vi "Convert Array from IH.vi"(1 "IH":T1) -> (0 "Array":u8[](array[numeric]))   [LabVIEW 2013, in "VRI.lvlib"]
uses:
  VRI.lvlib
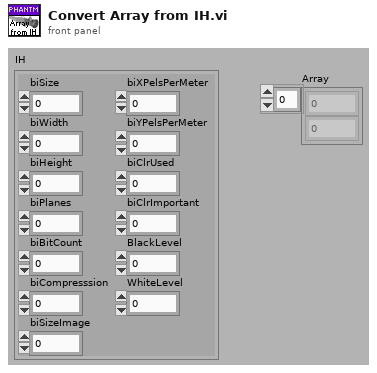
[diagram p1: front panel]
types:
  T1 = cluster{"biSize":u32, "biWidth":i32, "biHeight":i32, "biPlanes":u16, "biBitCount":u16, "biCompresssion":u32, "biSizeImage":u32, "biXPelsPerMeter":i32, "biYPelsPerMeter":i32, "biClrUsed":u32, "biClrImportant":u32, "BlackLevel":i32, "WhiteLevel":i32}
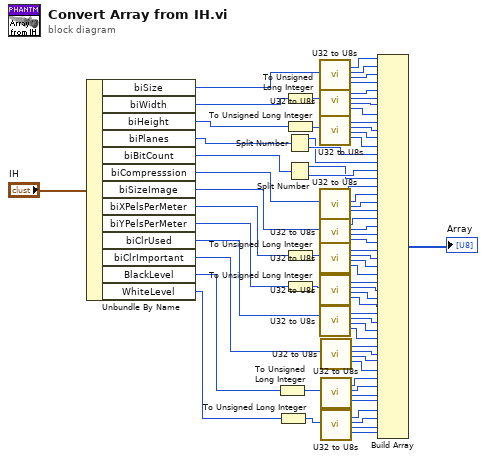
[diagram p0: block diagram]
diagram:
  n1 = Unbundle By Name("IH") -> ("biSize"=w14:u32, "biWidth"=w19:i32, "biHeight"=w26:i32, "biPlanes"=w31:u16, "biBitCount"=w34:u16, "biCompresssion"=w39:u32, "biSizeImage"=w48:u32, "biXPelsPerMeter"=w57:i32, "biYPelsPerMeter"=w58:i32, "biClrUsed"=w59:u32, "biClrImportant"=w60:u32, "BlackLevel"=w12:i32, "WhiteLevel"=w11:i32)
  n2 = To Unsigned Long Integer(number=w12) -> (unsigned 32bit integer=w10:u32)
  n3 = To Unsigned Long Integer(number=w11) -> (unsigned 32bit integer=w5:u32)
  n4 = To Unsigned Long Integer(number=w19) -> (unsigned 32bit integer=w25:u32)
  n5 = To Unsigned Long Integer(number=w26) -> (unsigned 32bit integer=w24:u32)
  n6 = Split Number(x=w31) -> (hi(x)=w32:u8, lo(x)=w33:u8)
  n7 = Split Number(x=w34) -> (hi(x)=w35:u8, lo(x)=w36:u8)
  n8 = To Unsigned Long Integer(number=w57) -> (unsigned 32bit integer=w37:u32)
  n9 = To Unsigned Long Integer(number=w58) -> (unsigned 32bit integer=w38:u32)
  n10 = call "U32 to U8s.vi"("U32"=w14) -> ("HiHi"=w15:u8, "Hi"=w16:u8, "Lo"=w17:u8, "LoLo"=w18:u8)  [unwired: 15 out]
  n11 = call "U32 to U8s.vi"("U32"=w25) -> ("HiHi"=w20:u8, "Hi"=w21:u8, "Lo"=w22:u8, "LoLo"=w23:u8)  [unwired: 15 out]
  n12 = call "U32 to U8s.vi"("U32"=w24) -> ("HiHi"=w27:u8, "Hi"=w28:u8, "Lo"=w29:u8, "LoLo"=w30:u8)  [unwired: 15 out]
  n13 = call "U32 to U8s.vi"("U32"=w39) -> ("HiHi"=w40:u8, "Hi"=w41:u8, "Lo"=w42:u8, "LoLo"=w43:u8)  [unwired: 15 out]
  n14 = call "U32 to U8s.vi"("U32"=w48) -> ("HiHi"=w44:u8, "Hi"=w45:u8, "Lo"=w46:u8, "LoLo"=w47:u8)  [unwired: 15 out]
  n15 = call "U32 to U8s.vi"("U32"=w37) -> ("HiHi"=w49:u8, "Hi"=w50:u8, "Lo"=w51:u8, "LoLo"=w52:u8)  [unwired: 15 out]
  n16 = call "U32 to U8s.vi"("U32"=w38) -> ("HiHi"=w53:u8, "Hi"=w54:u8, "Lo"=w55:u8, "LoLo"=w56:u8)  [unwired: 15 out]
  n17 = call "U32 to U8s.vi"("U32"=w59) -> ("HiHi"=w61:u8, "Hi"=w62:u8, "Lo"=w63:u8, "LoLo"=w64:u8)  [unwired: 15 out]
  n18 = call "U32 to U8s.vi"("U32"=w60) -> ("HiHi"=w65:u8, "Hi"=w66:u8, "Lo"=w67:u8, "LoLo"=w68:u8)  [unwired: 15 out]
  n19 = call "U32 to U8s.vi"("U32"=w10) -> ("HiHi"=w9:u8, "Hi"=w8:u8, "Lo"=w7:u8, "LoLo"=w6:u8)  [unwired: 15 out]
  n20 = call "U32 to U8s.vi"("U32"=w5) -> ("HiHi"=w4:u8, "Hi"=w3:u8, "Lo"=w2:u8, "LoLo"=w1:u8)  [unwired: 15 out]
  n21 = Build Array(w15, w16, w17, w18, w20, w21, w22, w23, w27, w28, w29, w30, w33, w32, w36, w35, w40, w41, w42, w43, w44, w45, w46, w47, w49, w50, w51, w52, w53, w54, w55, w56, w61, w62, w63, w64, w65, w66, w67, w68, w9, w8, w7, w6, w4, w3, w2, w1) -> (→"Array":u8[])
